vi "Motion_Initialize.vi"(8 "error in":errorcluster, 11 "TCP address:port (192.168.0.3:502)":string="192.168.0.3:502") -> (0 "error out":errorcluster, 3 "connection ID":refnum<k5>)   [LabVIEW 2010]
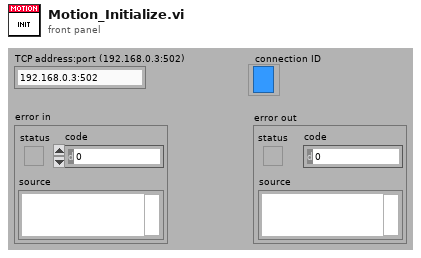
[diagram p1: front panel]
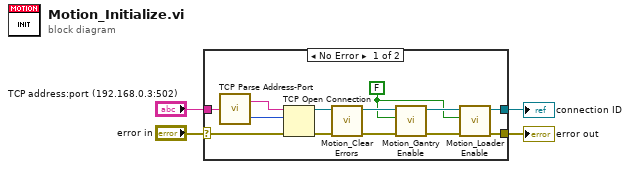
[diagram p0: block diagram]
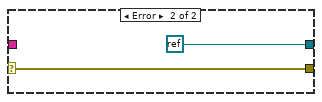
[diagram p2: hidden frame]
diagram:
  n1 = case shown="No Error" "error in" {
    selector: "error in" -> [w17 w18]
    tunnel: [w6 w18] -> w4
    tunnel: [w9 refnum<k0> refnum] -> w3
    tunnel: "TCP address:port (192.168.0.3:502)" -> [w14 _]
    frame No Error {
      w5 = FALSE
      n2 = call "TCP Parse Address-Port.vi"("TCP address:port"=w14) -> ("port"=w13:u16, "address"=w12:string)
      n3 = TCP Open Connection(address=w12, remote port or service name=w13, error in (no error)=w17) -> (connection ID=w15:refnum<k5>, error out=w16:errorcluster)  [unwired: 2 in]
      n4 = call "Motion_Clear Errors.vi"("error in (no error)"=w16, "TCP Connection Refnum in"=w15) -> ("error out"=w8:errorcluster, "TCP Connection Refnum (dup)"=w11:refnum<k5>)  [unwired: 8 in]
      n5 = call "Motion_Gantry Enable.vi"("error in (no error)"=w8, "Enable? (T)"=w5, "TCP Connection Refnum in"=w11) -> ("error out"=w7:errorcluster, "TCP Connection Refnum (dup)"=w10:refnum<k5>)  [unwired: 7 in]
      n6 = call "Motion_Loader Enable.vi"("error in (no error)"=w7, "Enable? (T)"=w5, "TCP Connection Refnum in"=w10) -> ("error out"=w6:errorcluster, "TCP Connection Refnum (dup)"=w9:refnum<k5>)  [unwired: 7 in]
    }
    frame Error {
    }
  }
  "error out" <- w4
  "connection ID" <- w3
